vi "adjustdacutil2div.vi"(6 "smaller":bool, 7 "bigger":bool, 8 "step":dbl, 9 "min dac":dbl, 10 "max dac":dbl, 11 "ori dac":dbl) -> (0 "new min":dbl, 1 "no need":bool, 2 "dac":dbl, 3 "new max":dbl)   [LabVIEW 2012]
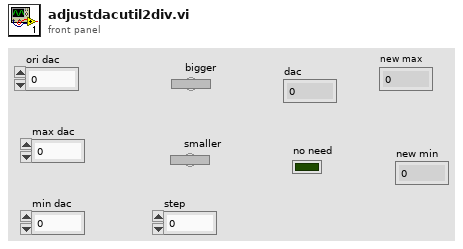
[diagram p1: front panel]
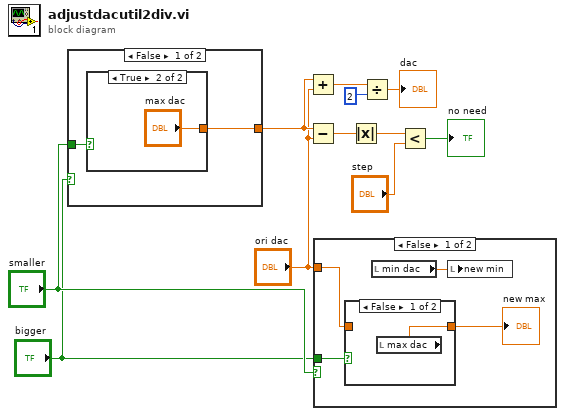
[diagram p0: block diagram]
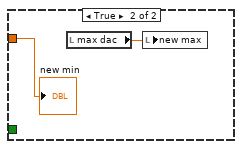
[diagram p3: hidden frame]
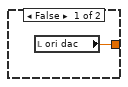
[diagram p4: hidden frame]
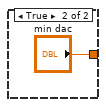
[diagram p5: hidden frame]
diagram:
  n1 = case shown="False" "bigger" {
    tunnel: [w12 "min dac"] -> w9
    tunnel: "smaller" -> [w13 _]
    frame False {
      n2 = case shown="True" w13 {
        tunnel: [w14 "max dac"] -> w12
        frame False {
          n3 = local read "ori dac"() -> (w14:dbl)
        }
        frame True {
        }
      }
    }
    frame True {
    }
  }
  n4 = Add(x=w9, y="ori dac") -> (x+y=w11:dbl)
  n5 = Subtract(x=w9, y="ori dac") -> (x-y=w8:dbl)
  n6 = case shown="False" "smaller" {
    tunnel: "bigger" -> [w20 _]
    tunnel: "ori dac" -> [w19 w24]
    frame False {
      n7 = case shown="False" w20 {
        tunnel: w19 -> [_ w22]
        tunnel: [w21 w22] -> w18
        frame False {
          n8 = local read "max dac"() -> (w21:dbl)
        }
        frame True {
        }
      }
      "new max" <- w18
      n9 = local read "min dac"() -> (w17:dbl)
      n10 = local write "new min"(w17) -> ()
    }
    frame True {
      n11 = local read "max dac"() -> (w23:dbl)
      n12 = local write "new max"(w23) -> ()
      "new min" <- w24
    }
  }
  n13 = Absolute Value(x=w8) -> (abs(x)=w7:dbl)
  n14 = Divide(x=w11, y=2) -> (x/y=→"dac":dbl)
  n15 = Less?(x=w7, y="step") -> (x < y?=→"no need":bool)
